vi "Update.vi"(6 "New Position":T1, 8 "error in (no error)":errorcluster, 9 "Pitch":sgl, 10 "Yaw":sgl, 11 "Player in":refnum<class "Player.lvclass">) -> (0 "error out":errorcluster, 3 "Player out":refnum<class "Player.lvclass">)   [LabVIEW 2015, in "Player.lvclass"]
uses:
  Player.lvclass
  3D Point.ctl
  Player.lvclass/Player.ctl
  3D Object/3D Object.lvclass/3D Object.ctl
  <vilib>/picture/3D Picture Control/Transformations/Get Translation.vi
  3D Object/3D Object.lvclass
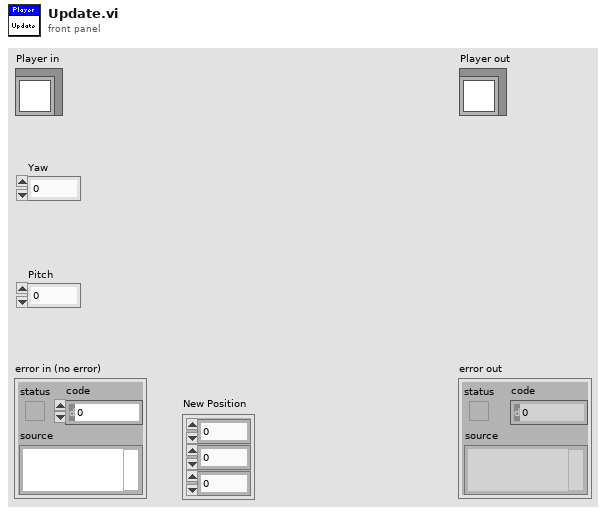
[diagram p1: front panel]
types:
  T1 = typedef "3D Point.ctl" = cluster{"X":sgl, "Y":sgl, "Z":sgl}
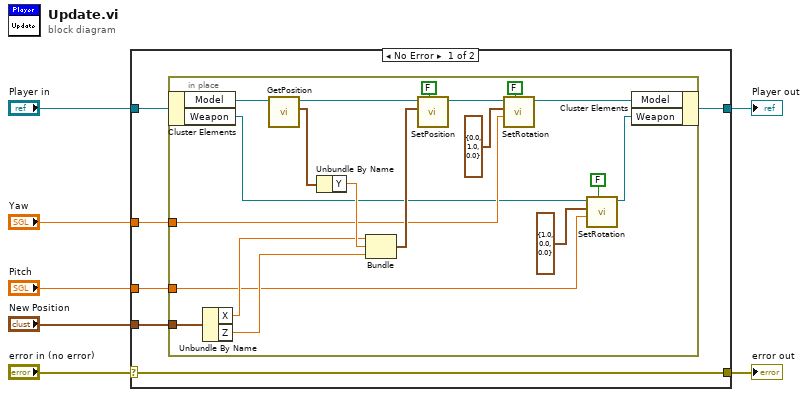
[diagram p0: block diagram]
diagram:
  n1 = case shown="No Error" "error in (no error)" {
    selector: "error in (no error)" -> [w13 w34]
    tunnel: [w13 w34] -> w6
    tunnel: [w11 w33] -> w4
    tunnel: "Player in" -> [w12 w33]
    tunnel: "New Position" -> [w10 _]
    tunnel: "Yaw" -> [w9 _]
    tunnel: "Pitch" -> [w8 _]
    frame No Error {
      n2 = in-place {
        in-place-border: w10 -> [w22]
        in-place-border: w9 -> [w18]
        in-place-border: w8 -> [w17]
        n3 = in-place-cluster #1(w12) -> ("Model"=w23:refnum<class "3D Object.lvclass">, "Weapon"=w15:refnum<class "3D Object.lvclass">)
        n4 = Unbundle By Name(w22) -> ("X"=w21:sgl, "Z"=w20:sgl)
        n5 = call "GetPosition.vi"("3D Object in"=w23) -> ("Position"=w30:cluster{"X":sgl, "Y":sgl, "Z":sgl}, "3D Object out"=w31:refnum<class "3D Object.lvclass">)  [unwired: 8 in, 1 out]
        n6 = Unbundle By Name(w30) -> ("Y"=w29:sgl)
        n7 = Bundle("X"=w21, "Y"=w29, "Z"=w20) -> (w19:cluster{"X":sgl, "Y":sgl, "Z":sgl})  [unwired: 1 in]
        n8 = call "SetPosition.vi"("Relative?"=FALSE, "Position"=w19, "3D Object in"=w31) -> ("3D Object out"=w28:refnum<class "3D Object.lvclass">)  [unwired: 7 in, 1 out]
        n9 = call "SetRotation.vi"("Relative?"=FALSE, "Angle"=w18, "Axis"=cluster{"X":sgl, "Y":sgl, "Z":sgl} {"X"=0.0, "Y"=1.0, "Z"=0.0}, "3D Object in"=w28) -> ("3D Object out"=w16:refnum<class "3D Object.lvclass">)  [unwired: 6 in, 1 out]
        n10 = call "SetRotation.vi"("Relative?"=FALSE, "Angle"=w17, "Axis"=cluster{"X":sgl, "Y":sgl, "Z":sgl} {"X"=1.0, "Y"=0.0, "Z"=0.0}, "3D Object in"=w15) -> ("3D Object out"=w14:refnum<class "3D Object.lvclass">)  [unwired: 6 in, 1 out]
        n11 = in-place-cluster #1("Model"=w16, "Weapon"=w14) -> (w11:refnum<class "Player.lvclass">)
      }
    }
    frame Error {
    }
  }
  "error out" <- w6
  "Player out" <- w4
